vi "MainFormClosing.vi"(11 "Caller":refnum<vi>) -> ()   [LabVIEW 2024]
panel:
  out "String":string
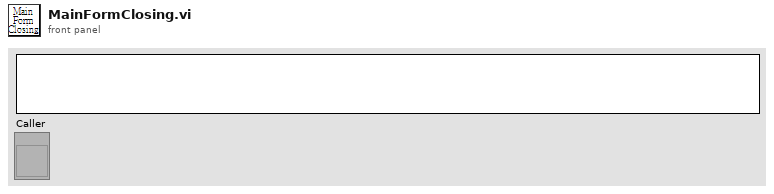
[diagram p1: front panel]
types:
  T1 = enum32{"Bad", "Idle", "Run top level", "Running"}
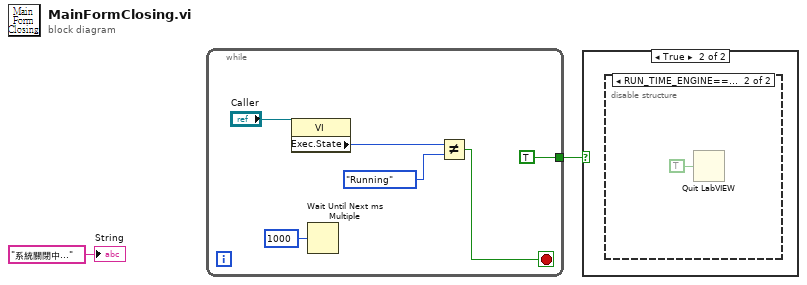
[diagram p0: block diagram]
diagram:
  n1 = while {
    tunnel: [TRUE] -> w1
    stop <- w4 stop-if-true
    n2 = property class="VI"(reference="Caller") -> ("Exec.State"=w5:T1)  [unwired: 1 in, 2 out]
    n3 = Wait Until Next ms Multiple(millisecond multiple=u32 1000) -> ()  [unwired: 1 out]
    n4 = Not Equal?(x=w5, y=T1."Running" ("Execution:State")) -> (x != y?=w4:bool)
  }
  n5 = case shown="True" w1 {
    frame False {
    }
    frame True {
      n6 = disable-structure shown="RUN_TIME_ENGINE==True" {
        frame condition #0 (active) {
        }
        frame condition #1 {
          n7 = Quit LabVIEW(quit? (T)=TRUE) -> ()
        }
      }
    }
  }
  "String" <- "系統關閉中..." ("String")
